vi "SF2_Get_Notifier_REF_Once.vi"() -> (3 "notifier ref out":refnum<notifier>, 4 "notification":T1)   [LabVIEW 2016]
uses:
  SF2_NotifyPacketTypeDef.ctl
  SF2_ActionTypeDef.ctl
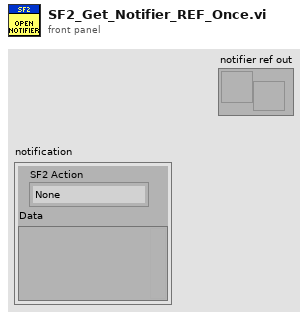
[diagram p1: front panel]
types:
  T1 = typedef "SF2_NotifyPacketTypeDef.ctl" = cluster{"SF2 Action":T2, "Data":variant}
  T2 = typedef "SF2_ActionTypeDef.ctl" = enum16{"None", "Halt", "Reset Buffer"}
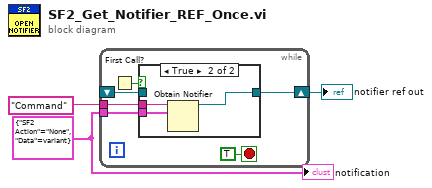
[diagram p0: block diagram]
diagram:
  w2 = T1 {"SF2 Action"=enum."None", "Data"=variant} ("notification")
  n1 = while {
    tunnel: "Command" ("name (unnamed)") -> [w9]
    tunnel: w2 -> [w8]
    shift-right: [w5] -> w1
    shift-left: _ -> [w4]
    stop <- TRUE stop-if-true
    n2 = First Call?() -> (First Call?: T/F=w7:bool)
    n3 = case shown="True" w7 {
      tunnel: w9 -> [_ w13]
      tunnel: w8 -> [_ w12]
      tunnel: [w10 w11] -> w5
      tunnel: w4 -> [w10 _]
      frame False {
      }
      frame True {
        n4 = Obtain Notifier(name (unnamed)=w13, notification data type=w12) -> (notifier out=w11:refnum<notifier>)  [unwired: 2 in, 2 out]
      }
    }
  }
  "notifier ref out" <- w1
  "notification" <- w2
